vi "Shutdown.vi"(8 "error in":errorcluster, 11 "DIG_IO in":refnum<class "DIG_IO.lvclass">) -> (0 "error out":errorcluster, 3 "DIG_IO out":refnum<class "DIG_IO.lvclass">)   [LabVIEW 2019, in "DIG_IO.lvlib" / "DIG_IO.lvclass"]
doc: "This routine performs a safe shutdown. It makes sure the digital outputs are all set to off before disconnecting from the IO device."
uses:
  Library/DIG_IO.lvclass
  builds/Instruments/Instruments.lvlibp/Library/Instruments.lvclass
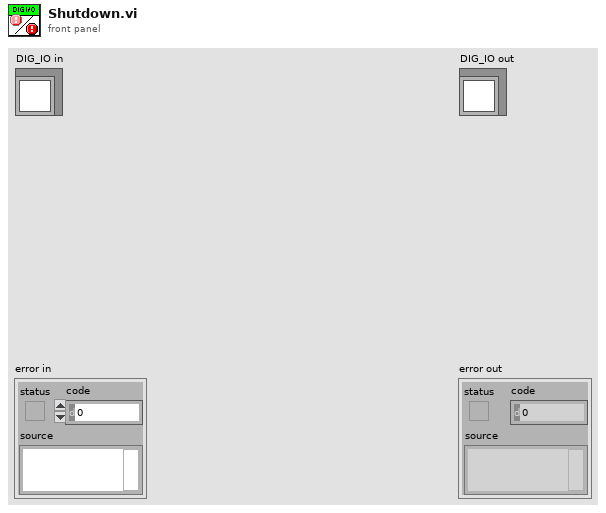
[diagram p1: front panel]
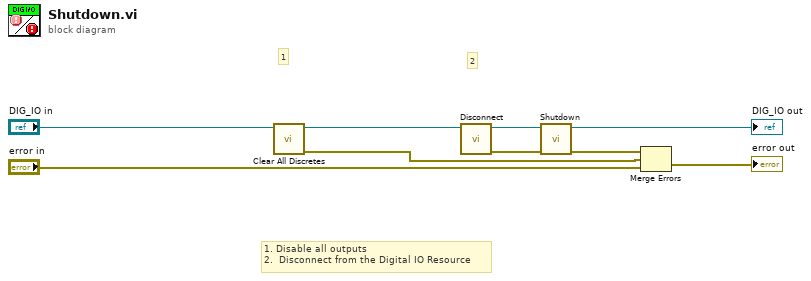
[diagram p0: block diagram]
diagram:
  # "1. Disable all outputs\n2.  Disconnect from the Digital IO Resource"
  # "2"
  # "1"
  n1 = call-dynamic "Clear All Discretes.vi"("DIG_IO in"="DIG_IO in") -> ("error out"=w1:errorcluster, "DIG_IO out"=w2:refnum<class "DIG_IO.lvclass">)  [unwired: 9 in]
  n2 = call-dynamic "Disconnect.vi"("DIG_IO in"=w2) -> ("error out"=w5:errorcluster, "DIG_IO out"=w7:refnum<class "DIG_IO.lvclass">)  [unwired: 9 in]
  n3 = call-parent "Shutdown.vi"("error in"=w5, "Instruments in"=w7) -> ("error out"=w4:errorcluster, "Instruments out"=→"DIG_IO out":refnum<class "DIG_IO.lvclass">)  [unwired: 8 in]
  n4 = Merge Errors(w4, w1, "error in") -> (→"error out":errorcluster)
